vi "Switch Configuration - Scan List Generation Mode Init.vi"(8 "error in (no error)":errorcluster, 11 "Switch Config UI Data In":T1 {"Switch Config Page Item Ref" format="%.0x"}) -> (0 "error out":errorcluster, 3 "Switch Config UI Data Out":T1 {"Switch Config Page Item Ref" format="%.0x"})   [LabVIEW 2015, in "DMM-SWITCH-ScanList System Explorer.lvlib"]
doc: "Enable/Disable controls and indicators depending on Scan List Generation Mode (Manual/Automatic)"
uses:
  DMM-SWITCH-ScanList System Explorer.lvlib
  Configuration Controls/Switch Config VI UI Data.ctl
  Configuration Controls/Switch Config VI UI Ctrl Values.ctl
  Configuration Controls/Switch Config VI UI Ctrl References.ctl
  <instrlib>/niSwitch/niSwitch.LLB/niSwitch Topologies.ctl
  <vilib>/NI Veristand/Custom Device API/Custom Device Item Ref.ctl
  <vilib>/NI Veristand/Custom Device API/Custom Device API.lvlib
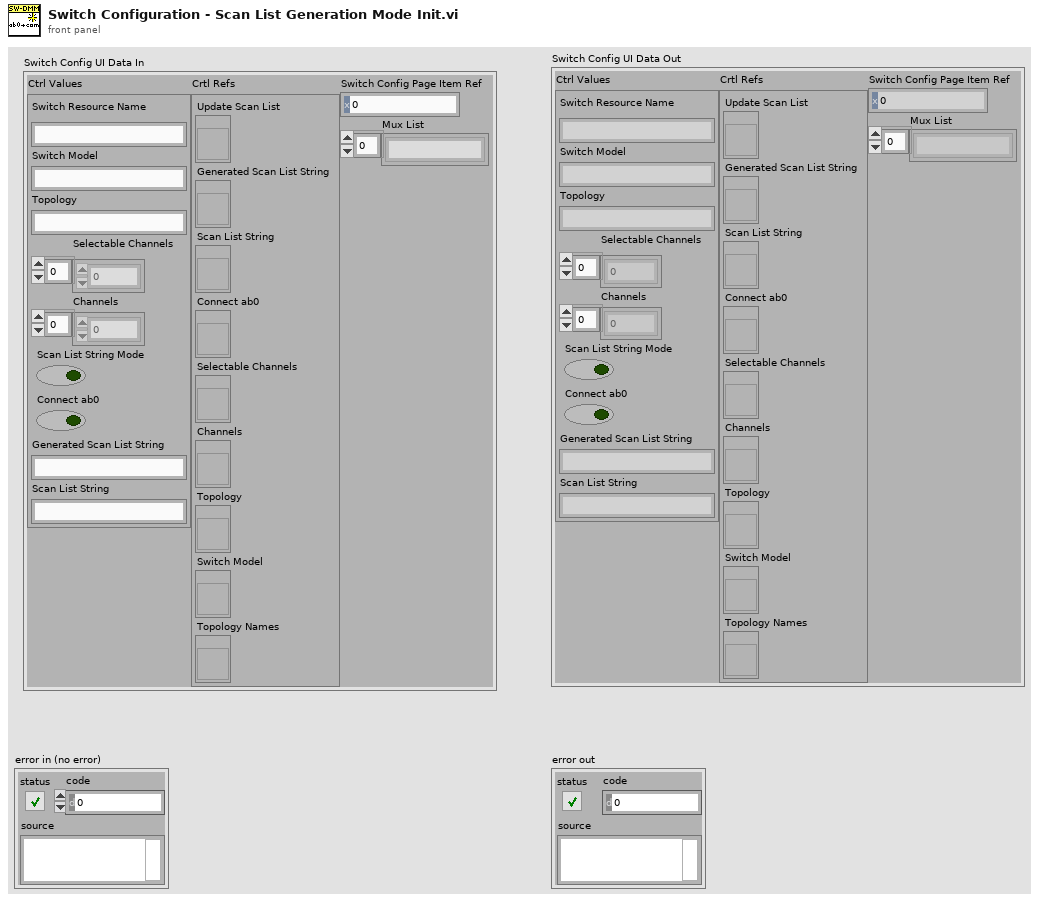
[diagram p1: front panel]
types:
  T1 = typedef "DMM-SWITCH-ScanList System Explorer.lvlib/Switch Config VI UI Data.ctl" = cluster{"Ctrl Values":T2, "Crtl Refs":T3, "Switch Config Page Item Ref":T4, "Mux List":string[]}
  T2 = typedef "DMM-SWITCH-ScanList System Explorer.lvlib/Switch Config VI UI Ctrl Values.ctl" = cluster{"Switch Resource Name":string, "Switch Model":string, "Topology":string, "Selectable Channels":i32[], "Channels":i32[], "Scan List String Mode":bool, "Connect ab0":bool, "Generated Scan List String":string, "Scan List String":string}
  T3 = typedef "DMM-SWITCH-ScanList System Explorer.lvlib/Switch Config VI UI Ctrl References.ctl" = cluster{"Update Scan List":refnum<vi>, "Generated Scan List String":refnum<vi>, "Scan List String":refnum<vi>, "Connect ab0":refnum<vi>, "Selectable Channels":refnum<vi>, "Channels":refnum<vi>, "Topology":refnum<vi>, "Switch Model":refnum<vi>, "Topology Names":refnum<vi>}
  T4 = typedef "Custom Device API.lvlib/Custom Device Item Ref.ctl" = u64
  T5 = enum8{"Enabled", "Disabled", "Disabled and Grayed Out"}
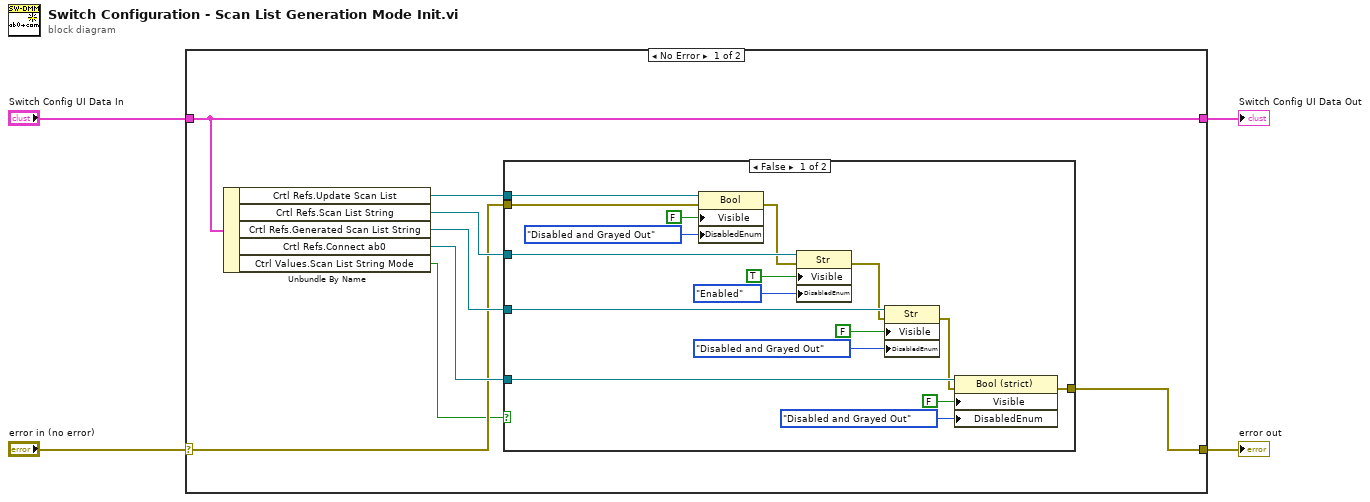
[diagram p0: block diagram]
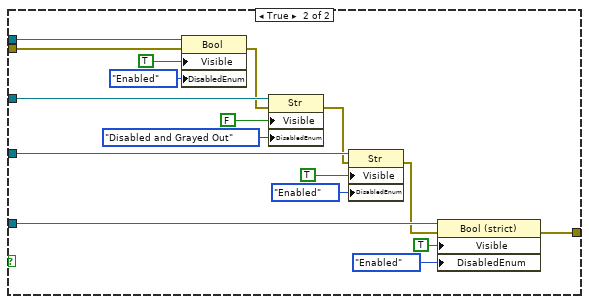
[diagram p2: hidden frame]
diagram:
  n1 = case shown="No Error" "error in (no error)" {
    selector: "error in (no error)" -> [w7 w48]
    tunnel: [w12 w48] -> w4
    tunnel: "Switch Config UI Data In" -> [w5 w47]
    tunnel: [w5 w47] -> w1
    frame No Error {
      n2 = Unbundle By Name(w5) -> ("Crtl Refs.Update Scan List"=w11:refnum<vi>, "Crtl Refs.Scan List String"=w10:refnum<vi>, "Crtl Refs.Generated Scan List String"=w9:refnum<vi>, "Crtl Refs.Connect ab0"=w8:refnum<vi>, "Ctrl Values.Scan List String Mode"=w6:bool)
      n3 = case shown="False" w6 {
        tunnel: w10 -> [w29 w46]
        tunnel: w9 -> [w24 w41]
        tunnel: w8 -> [w21 w38]
        tunnel: w7 -> [w18 w34]
        tunnel: w11 -> [w19 w35]
        tunnel: [w13 w30] -> w12
        frame False {
          n4 = property class="Bool"(reference=w19, error in=w18, "Visible"=FALSE, "DisabledEnum"=T5."Disabled and Grayed Out" ("Disabled")) -> (error out=w16:errorcluster)  [unwired: 1 out]
          n5 = property class="Str"(reference=w29, error in=w16, "Visible"=TRUE, "DisabledEnum"=T5."Enabled" ("Disabled")) -> (error out=w15:errorcluster)  [unwired: 1 out]
          n6 = property class="Str"(reference=w24, error in=w15, "Visible"=FALSE, "DisabledEnum"=T5."Disabled and Grayed Out" ("Disabled")) -> (error out=w14:errorcluster)  [unwired: 1 out]
          n7 = property class="Bool (strict)"(reference=w21, error in=w14, "Visible"=FALSE, "DisabledEnum"=T5."Disabled and Grayed Out" ("Disabled")) -> (error out=w13:errorcluster)  [unwired: 1 out]
        }
        frame True {
          n8 = property class="Bool"(reference=w35, error in=w34, "Visible"=TRUE, "DisabledEnum"=T5."Enabled" ("Disabled")) -> (error out=w33:errorcluster)  [unwired: 1 out]
          n9 = property class="Str"(reference=w46, error in=w33, "Visible"=FALSE, "DisabledEnum"=T5."Disabled and Grayed Out" ("Disabled")) -> (error out=w32:errorcluster)  [unwired: 1 out]
          n10 = property class="Str"(reference=w41, error in=w32, "Visible"=TRUE, "DisabledEnum"=T5."Enabled" ("Disabled")) -> (error out=w31:errorcluster)  [unwired: 1 out]
          n11 = property class="Bool (strict)"(reference=w38, error in=w31, "Visible"=TRUE, "DisabledEnum"=T5."Enabled" ("Disabled")) -> (error out=w30:errorcluster)  [unwired: 1 out]
        }
      }
    }
    frame Error {
    }
  }
  "error out" <- w4
  "Switch Config UI Data Out" <- w1
